vi "Sucesion 3.vi"() -> ()   [LabVIEW 2017]
panel:
  out "Iteración":i64
  out "Número":i64
  # "SUCESIÓN 3"
  # "Cecilia Nuñez\n  11541028"
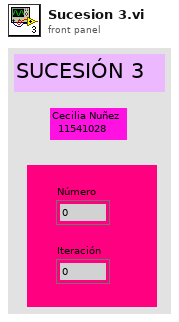
[diagram p1: front panel]
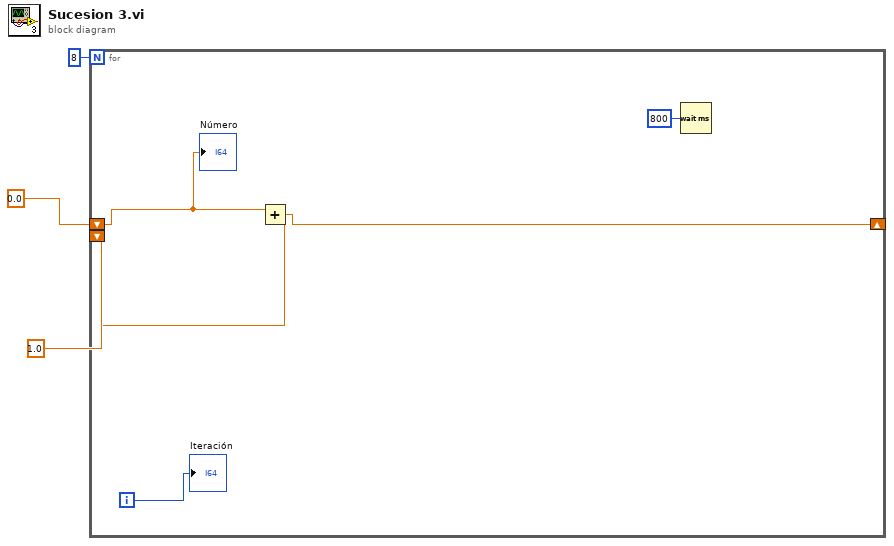
[diagram p0: block diagram]
diagram:
  n1 = for {
    N: 8 -> [_]
    shift-right: [w6] -> _
    shift-left: 0.0 -> [w4]
    shift-left: 1.0 -> [w5]
    i -> [w8]
    n2 = Add(x=w4, y=w5) -> (x+y=w6:dbl)
    n3 = Wait (ms)(milliseconds to wait=u32 800) -> ()  [unwired: 1 out]
    "Iteración" <- w8
    "Número" <- w4
  }
